vi "Example- Run Engine Simulation.vi"() -> ()   [LabVIEW 2013]
uses:
  API/APU/APU.lvclass
  API/APU/Setup APU 1.3.vi
  API/APU/Write APU 1.3 Speed.vi
  API/APU/Read APU 1.3 Position.vi
  API/Engine Simulation Session.lvclass
panel:
  out "found":bool
  out "crank angle":dbl
  out "cycle angle":dbl
  in  "speed (RPM)":dbl
  in  "stop":bool
  in  "device address":string="RIO0"
  out "error out":errorcluster
  in  "bitfile":path
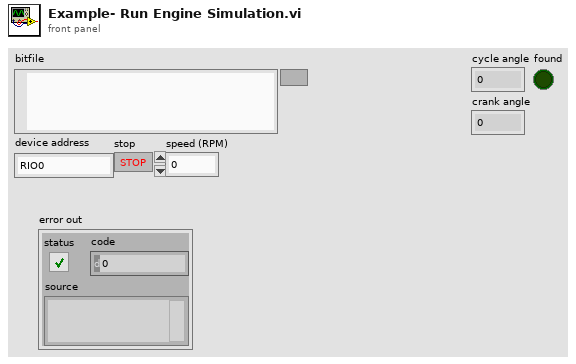
[diagram p1: front panel]
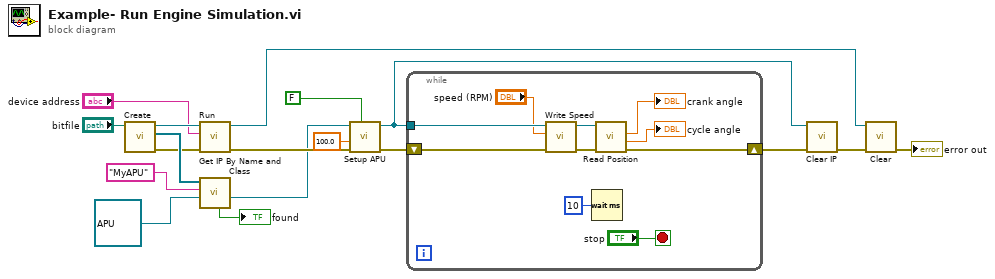
[diagram p0: block diagram]
diagram:
  n1 = call "Create.vi"("bitfile"="bitfile") -> ("error out"=w14:errorcluster, "IPs"=w17:refnum<class "Engine Simulation IP.lvclass">[], "Engine Simulation Session out"=w16:refnum<class "Engine Simulation Session.lvclass">)  [unwired: 6 in, 2 out]
  n2 = call "Run.vi"("error in (no error)"=w14, "device address"="device address", "Engine Simulation Session in"=w16) -> ("error out"=w13:errorcluster, "Engine Simulation Session out"=w8:refnum<class "Engine Simulation Session.lvclass">)  [unwired: 7 in]
  n3 = call-dynamic "Get IP By Name and Class.vi"("class"=refnum<class "APU.lvclass"> refnum ("APU.lvclass"), "name"="MyAPU", "IP"=w17) -> ("IP"=w3:refnum<class "APU.lvclass">, "found"=→"found":bool)  [unwired: 7 in]
  n4 = call-poly "Setup APU.vi"("enable acceleration (F)"=FALSE ("Enable Acceleration"), "error in (no error)"=w13, "start position (deg) (0)"=100.0, "APU in"=w3) -> ("error out"=w12:errorcluster, "APU out"=w6:refnum<class "APU.lvclass">)  [unwired: 6 in]
  n5 = while {
    shift-right: [w24] -> w7
    shift-left: w12 -> [w27]
    tunnel: w6 -> [w28]
    stop <- "stop" stop-if-true
    n6 = call-poly "Write Speed.vi"("error in (no error)"=w27, "speed (RPM)"="speed (RPM)", "APU in"=w28) -> ("error out"=w25:errorcluster, "APU out"=w26:refnum<class "APU.lvclass">)  [unwired: 7 in]
    n7 = Wait (ms)(milliseconds to wait=u32 10) -> ()  [unwired: 1 out]
    n8 = call-poly "Read Position.vi"("error in (no error)"=w25, "APU in"=w26) -> ("error out"=w24:errorcluster, "cycle angle"=→"cycle angle":dbl, "crank angle"=→"crank angle":dbl)  [unwired: 6 in, 1 out]
  }
  n9 = call-dynamic "Clear IP.vi"("error in (no error)"=w7, "APU in"=w6) -> ("error out"=w5:errorcluster)  [unwired: 9 in]
  n10 = call "Clear.vi"("error in (no error)"=w5, "Engine Simulation Session"=w8) -> ("error out"=→"error out":errorcluster)  [unwired: 9 in]
